vi "Benchmark Cleanup.vi"(8 "error in (no error)":errorcluster, 11 "CIFCorePlugin in":refnum<class "CIFCorePlugin.lvclass">) -> (0 "error out":errorcluster, 3 "CIFCorePlugin out":refnum<class "CIFCorePlugin.lvclass">)   [LabVIEW 2021, in "CIFCorePlugin.lvclass"]
uses:
  CIFCorePlugin.lvclass
  CIFCorePlugin.lvclass/CIFCorePlugin.ctl
  <vilib>/CIF Foundation/CIF Utilities/Statistics/I64/Stats_I64_CIF_U.lvclass/Stats_I64_CIF_U.ctl
  Accessors/Timestamps/Read Cleanup TS.vi
  <vilib>/CIF Foundation/CIF Utilities/Statistics/I64/X1 minus X0.vi/dfabcf33-0dbc-4041-80a5-3dc0c86d2989.vi
  <vilib>/CIF Foundation/CIF Utilities/Time/System Time/LabVIEW Time to TAI Time.vi
  <vilib>/CIF Foundation/CIF Utilities/Statistics/I64/X1 minus X0.vi/dfabcf33-0dbc-4041-80a5-3dc0c86d2989.vi/9eb60a9a-770f-4d2d-8b3f-8465c267ecc9.vi
  <vilib>/CIF Foundation/CIF Utilities/Time/Time_CIF_U.lvlib
  <vilib>/CIF Foundation/CIF Utilities/Statistics/I64/Stats_I64_CIF_U.lvclass
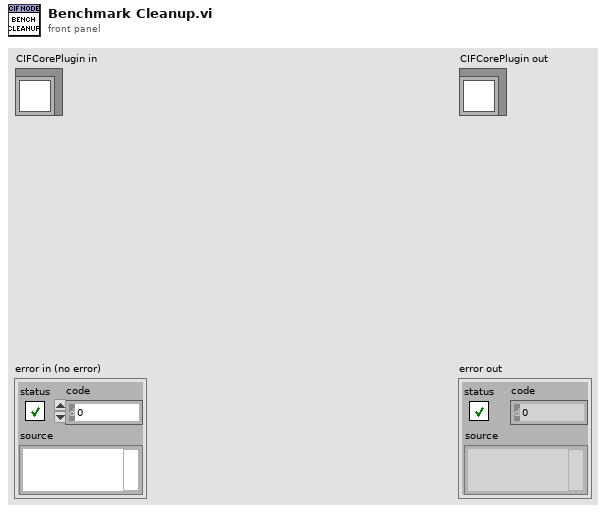
[diagram p1: front panel]
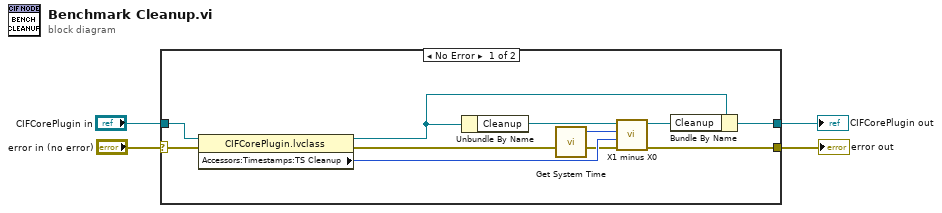
[diagram p0: block diagram]
diagram:
  n1 = case shown="No Error" "error in (no error)" {
    selector: "error in (no error)" -> [w11 w16]
    tunnel: [w14 w16] -> w1
    tunnel: [w8 w15] -> w2
    tunnel: "CIFCorePlugin in" -> [w13 w15]
    frame No Error {
      n2 = property class="CIFCorePlugin.lvclass"(reference=w13, error in=w11) -> (reference out=w9:refnum<class "CIFCorePlugin.lvclass">, error out=w10:errorcluster, "Accessors:Timestamps:TS Cleanup"=w12:i64)
      n3 = Unbundle By Name(w9) -> ("Cleanup"=w6:refnum<class "Stats_I64_CIF_U.lvclass">)
      n4 = call <vilib>:"Get System Time.vi"() -> ("Time (ns)"=w7:i64)  [unwired: 5 in]
      n5 = call <vilib>:"X1 minus X0.vi"("error in (no error)"=w10, "X0"=w12, "X1"=w7, "Stats_I64_CIF_U in"=w6) -> ("error out"=w14:errorcluster, "Stats_I64_CIF_U out"=w5:refnum<class "Stats_I64_CIF_U.lvclass">)  [unwired: 6 in]
      n6 = Bundle By Name(cluster=w9, "Cleanup"=w5) -> (w8:refnum<class "CIFCorePlugin.lvclass">)
    }
    frame Error {
    }
  }
  "error out" <- w1
  "CIFCorePlugin out" <- w2
